vi "Write String Var in.vi"(2 "Tag IN":string, 3 "错误输入（无错误）":errorcluster, 4 "String Var in":string, 5 "Ds PLCTags IN":T1[](array[typedef])) -> (0 "error out":errorcluster, 1 "Ds PLCTags OUT":T1[](array[typedef]))   [LabVIEW 2014]
uses:
  DataSocket_Tags.ctl
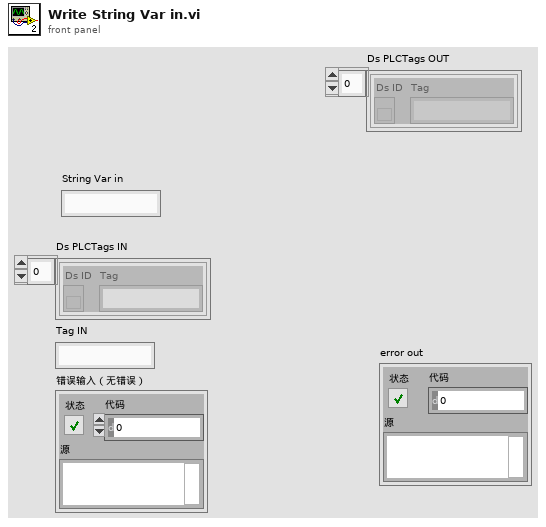
[diagram p1: front panel]
types:
  T1 = typedef "DataSocket_Tags.ctl" = cluster{"Ds ID":refnum<k13>, "Tag":string}
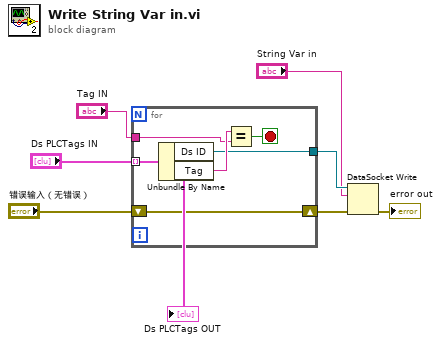
[diagram p0: block diagram]
diagram:
  n1 = for {
    tunnel: "Ds PLCTags IN" -> [w13] mode=indexing
    tunnel: "Tag IN" -> [w11]
    tunnel: [w9] -> w3
    shift-right: [w8] -> w2
    shift-left: "错误输入（无错误）" -> [w8]
    stop <- w10 stop-if-true
    n2 = Unbundle By Name(w13) -> ("Ds ID"=w9:refnum<k13>, "Tag"=w12:string)
    n3 = Equal?(x=w12, y=w11) -> (x = y?=w10:bool)
  }
  n4 = DataSocket Write(8:w2, 10:"String Var in", 11:w3) -> (0:→"error out":errorcluster)  [unwired: 1 in, 2 out]
  "Ds PLCTags OUT" <- "Ds PLCTags IN"
